vi "Is Supported Output.vi"(2 "Ctl Refnum":refnum<vi>) -> (7 "Type":T1, 9 "Supported":bool)   [LabVIEW 2015, in "CallVIStep.lvclass"]
uses:
  CallVIStep.lvclass
  Step/OUTPUT_DATA_TYPE.ctl
  Step.lvclass
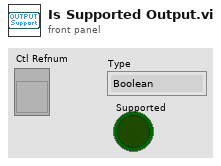
[diagram p1: front panel]
types:
  T1 = typedef "Step.lvclass/OUTPUT_DATA_TYPE.ctl" = enum16{"Boolean", "String", "Numeric", "Other"}
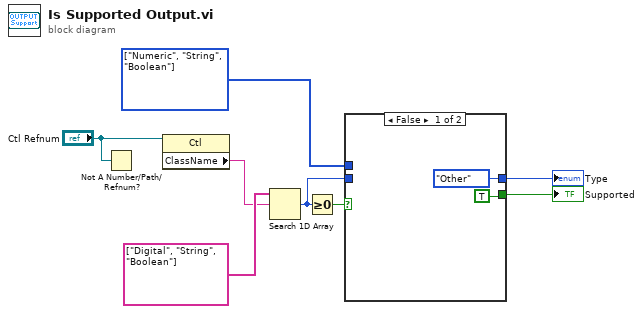
[diagram p0: block diagram]
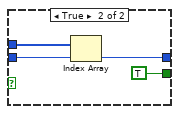
[diagram p2: hidden frame]
diagram:
  w4 = T1[] [enum."Numeric", enum."String", enum."Boolean"] items=["Boolean", "String", "Numeric", "Other"]
  n1 = Not A Number/Path/Refnum?(number/path/refnum="Ctl Refnum") -> ()  [unwired: 1 out]
  n2 = property class="Ctl"(reference="Ctl Refnum") -> ("ClassName"=w6:string)  [unwired: 1 in, 2 out]
  n3 = Search 1D Array(1D array=string[] ["Digital", "String", "Boolean"] ("Strings []"), element=w6) -> (index of element=w3:i32)  [unwired: 1 in]
  n4 = Greater Or Equal To 0?(x=w3) -> (x >= 0?=w5:bool)
  n5 = case shown="False" w5 {
    tunnel: w4 -> [_ w14]
    tunnel: w3 -> [_ w13]
    tunnel: [OUTPUT_DATA_TYPE."Other" ("Type") w12] -> w2
    tunnel: [TRUE TRUE] -> w1
    frame False {
    }
    frame True {
      n6 = Index Array(array=w14, index=w13) -> (element=w12:T1)
    }
  }
  "Supported" <- w1
  "Type" <- w2
